vi "Parse Step Status Response.vi"(8 "error in (no error)":errorcluster, 11 "Step Status":string[](array[string])) -> (0 "error out":errorcluster, 3 "Step Status":T1)   [LabVIEW 2018, in "F4T.lvlib" / "F4T.lvclass"]
uses:
  F4T.lvclass
  PPLs/Temp Chamber/Parent/Temp Chamber.lvlibp/Custom Controls/Step Status.ctl
  PPLs/Temp Chamber/Parent/Temp Chamber.lvlibp/Custom Controls/Step Type.ctl
  PPLs/Temp Chamber/Parent/Temp Chamber.lvlibp/Temp Chamber.lvclass
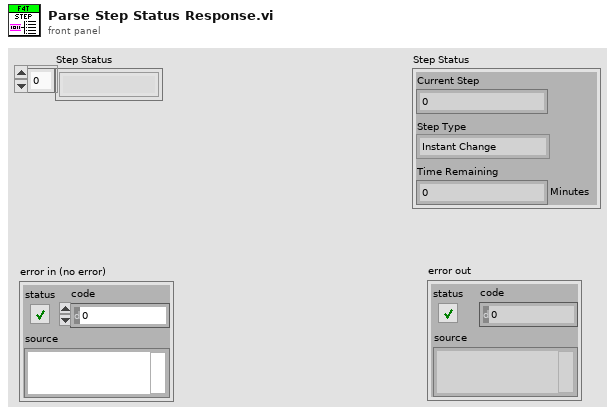
[diagram p1: front panel]
types:
  T1 = typedef "Temp Chamber.lvlibp/Temp Chamber.lvclass/Step Status.ctl" = cluster{"Current Step":u32, "Step Type":T2, "Time Remaining":u32}
  T2 = typedef "Temp Chamber.lvlibp/Temp Chamber.lvclass/Step Type.ctl" = enum16{"Instant Change", "Wait For", "Jump", "Soak", "Ramp Rate", "Ramp Time", "End", "Other"}
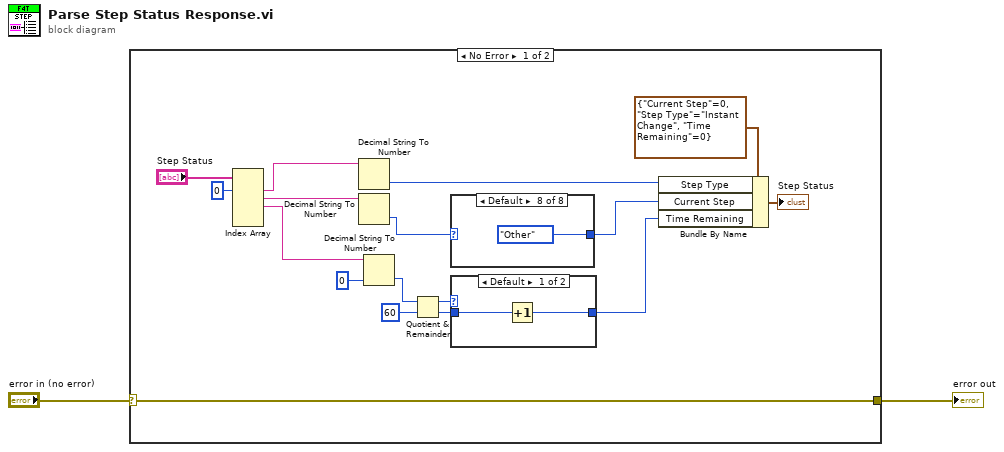
[diagram p0: block diagram]
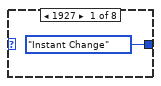
[diagram p3: hidden frame]
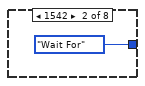
[diagram p4: hidden frame]
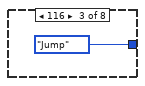
[diagram p5: hidden frame]
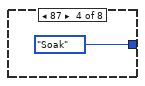
[diagram p6: hidden frame]
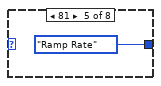
[diagram p7: hidden frame]
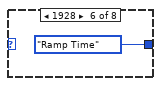
[diagram p8: hidden frame]
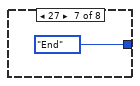
[diagram p9: hidden frame]
diagram:
  n1 = case shown="No Error" "error in (no error)" {
    selector: "error in (no error)" -> [w12 w31]
    tunnel: [w12 w31] -> w1
    frame No Error {
      n2 = Index Array(array="Step Status", index #1=0 ("index")) -> (element #1=w18:string, element #2=w16:string, element #3=w14:string)  [unwired: 4 in, 2 out]
      n3 = Decimal String To Number(string=w18) -> (number=w17:i32)  [unwired: 2 in, 1 out]
      n4 = Decimal String To Number(string=w16) -> (number=w15:i32)  [unwired: 2 in, 1 out]
      n5 = Decimal String To Number(string=w14, default (0L)=u32 0) -> (number=w8:u32)  [unwired: 1 in, 1 out]
      n6 = Quotient & Remainder(x=w8, y=u32 60) -> (x-y*floor(x/y)=w6:u32, floor(x/y)=w5:u32)
      n7 = case shown="Default" w15 {
        tunnel: [Step_Type."Instant Change" ("Step Type") Step_Type."Wait For" ("Step Type") Step_Type."Jump" ("Step Type") Step_Type."Soak" ("Step Type") Step_Type."Ramp Rate" ("Step Type") Step_Type."Ramp Time" ("Step Type") Step_Type."End" ("Step Type") Step_Type."Other" ("Step Type")] -> w3
        frame 1927 {
        }
        frame 1542 {
        }
        frame 116 {
        }
        frame 87 {
        }
        frame 81 {
        }
        frame 1928 {
        }
        frame 27 {
        }
        frame Default {
        }
      }
      n8 = case shown="Default" w6 {
        tunnel: w5 -> [w21 w22]
        tunnel: [w20 w22] -> w4
        frame Default {
          n9 = Increment(x=w21) -> (x+1=w20:u32)
        }
        frame 0 {
        }
      }
      n10 = Bundle By Name(cluster=T1 {"Current Step"=0, "Step Type"=enum."Instant Change", "Time Remaining"=0} ("Step Status"), "Step Type"=w17, "Current Step"=w3, "Time Remaining"=w4) -> (→"Step Status":T1)
    }
    frame Error {
    }
  }
  "error out" <- w1
